vi "Main Display Console.vi"(8 "error in (no error)":errorcluster, 11 "Module_Refs":T2={"ModuleName"=enum."Controller", "Queue"=refnum, "user event"=refnum, "VI Refnum"=refnum, "ShowFP"=FALSE, "StatesTracking Enabled"=FALSE}) -> (0 "error out":errorcluster)   [LabVIEW 2019, in "DisplayConsole.lvlib"]
doc: "Main Module Template of the architecture. Use this as a template to integrate new independent processes into your application."
uses:
  DisplayConsole.lvlib
  Architecture/Typedefs/Enum_Module_Name.ctl
  Architecture/Architecture.lvlib
  Architecture/Typedefs/Message.ctl
  Architecture/Typedefs/Module References.ctl
  Typedefs/State Machine Data.ctl
  Architecture/Typedefs/Application Configuration.ctl
  Typedefs/Config.ctl
  Architecture/Modules/Module Template/SubVIs/Module Template Configuraton Extractor API.vi
  Architecture/Modules/Module Template/Typedefs/Config.ctl
  Architecture/Modules/Module Template/Module Template.lvlib
panel:
  in  "Display Console":T1
  in  "Stop App":bool
  out "Message":string
  in  "Stop Module":bool
  # "#Architecture\n\nPlace inside this box all visible data."
  # "DISPLAY CONSOLE"
  # "[Covers: SI1]"
  # "[Covers: UI3]"
  # "[Covers: UI1]"
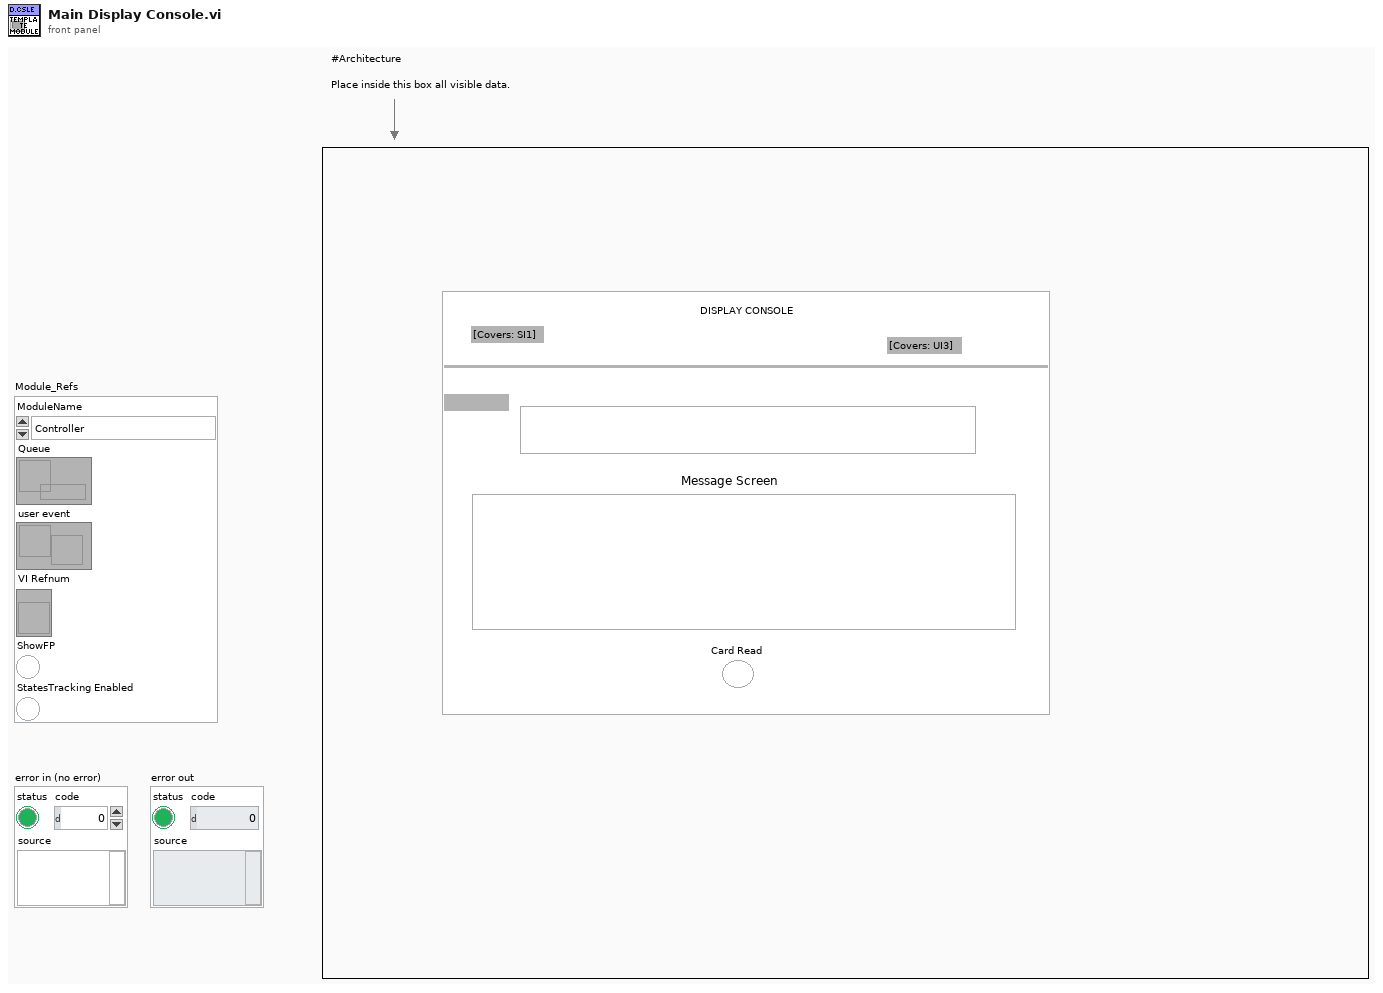
[diagram p1: front panel]
types:
  T1 = cluster{"Current Transaction":string, "Message Screen":string, "Card Read":bool}
  T2 = typedef "Architecture.lvlib/Module References.ctl" = cluster{"ModuleName":T3, "Queue":refnum<queue>, "user event":refnum<user-event>, "VI Refnum":refnum<vi>, "ShowFP":bool, "StatesTracking Enabled":bool}
  T3 = typedef "Architecture.lvlib/Enum_Module_Name.ctl" = enum16{"Configuration", "Error_Handler", "Log", "Database", "Controller", "User Console", "Display Console", "Sensor Interface"}
  T4 = typedef "DisplayConsole.lvlib/State Machine Data.ctl" = cluster{"Module_Refs":T2, "Response Data":variant, "Module Template Config":T5}
  T5 = typedef "DisplayConsole.lvlib/Config.ctl" = cluster{"Module Enabled":bool}
  T6 = enum32{"Invalid", "Standard", "Closed", "Hidden", "Minimized", "Maximized"}
  T7 = typedef "Architecture.lvlib/Module Template.lvlib/Config.ctl" = cluster{"Module Enabled":bool}
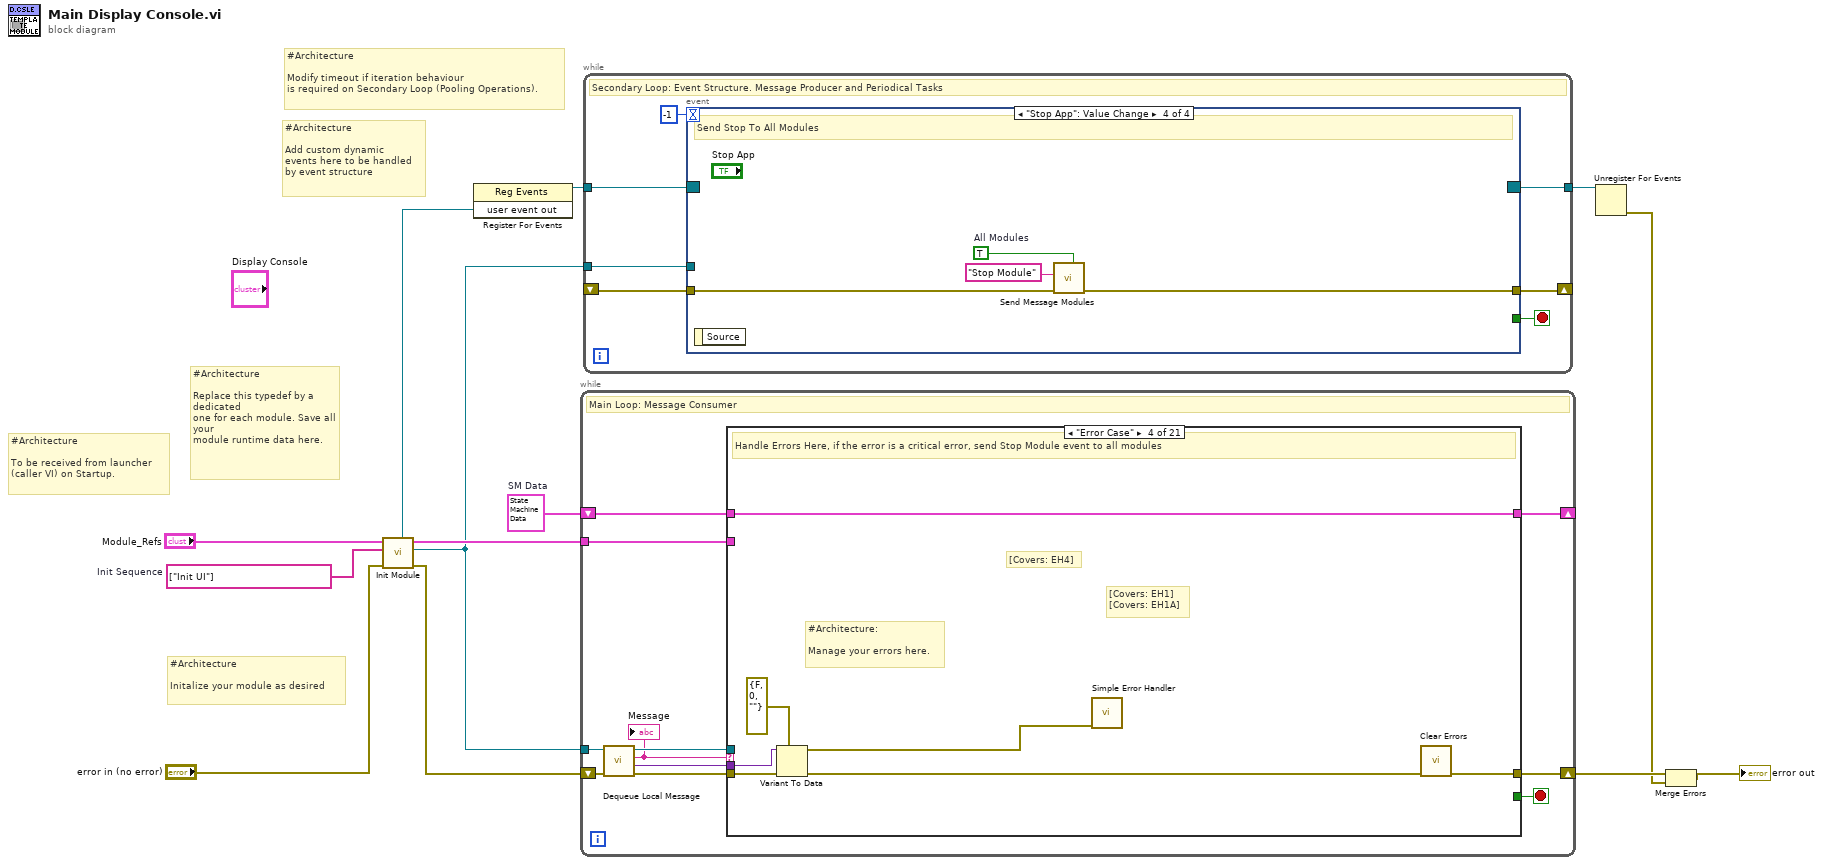
[diagram p0: block diagram]
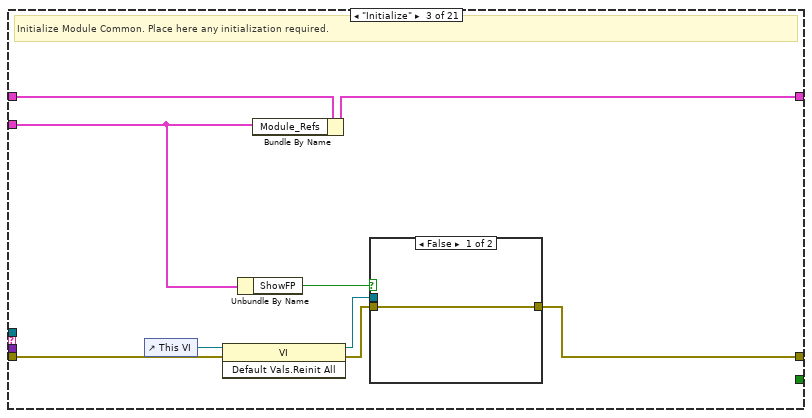
[diagram p4: hidden frame]
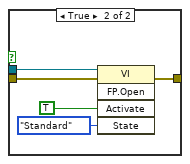
[diagram p5: hidden frame]
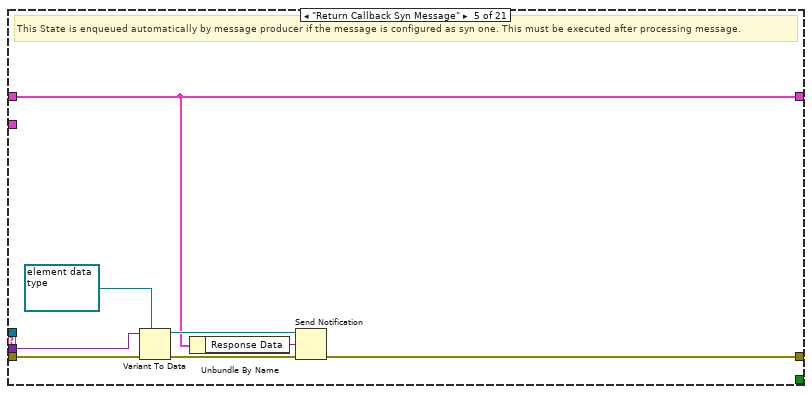
[diagram p6: hidden frame]
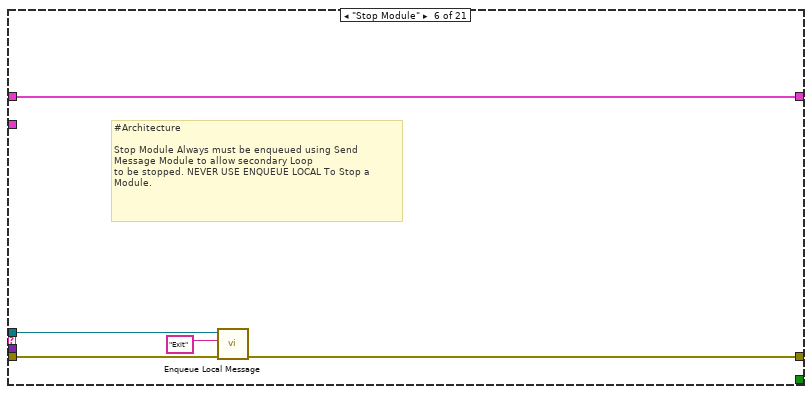
[diagram p7: hidden frame]
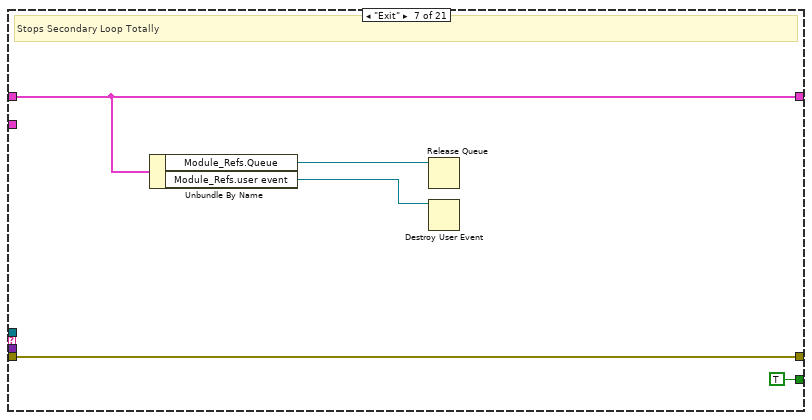
[diagram p8: hidden frame]
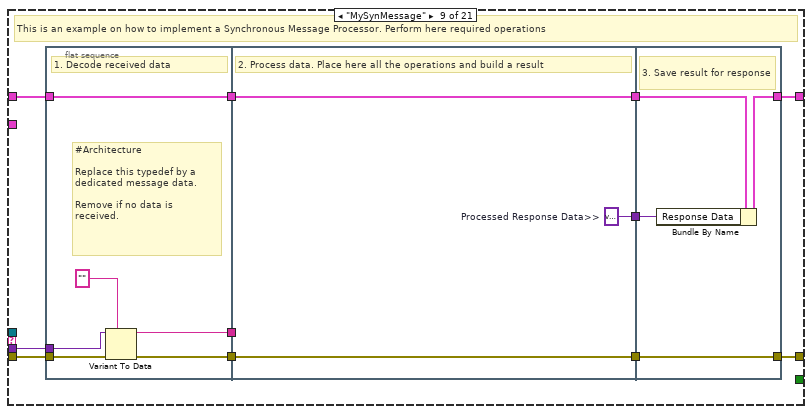
[diagram p10: hidden frame]
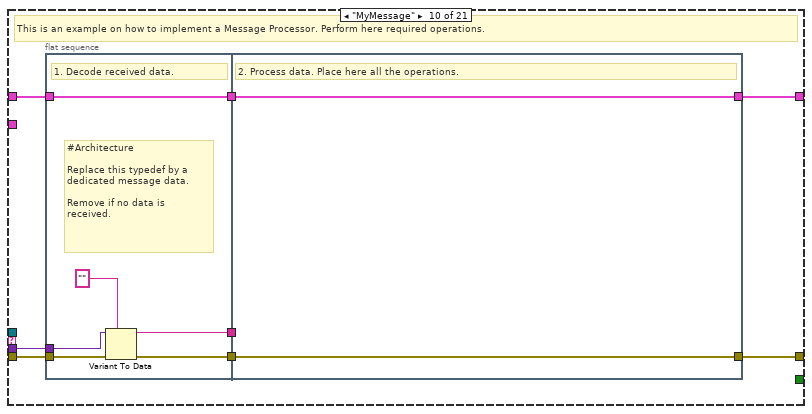
[diagram p11: hidden frame]
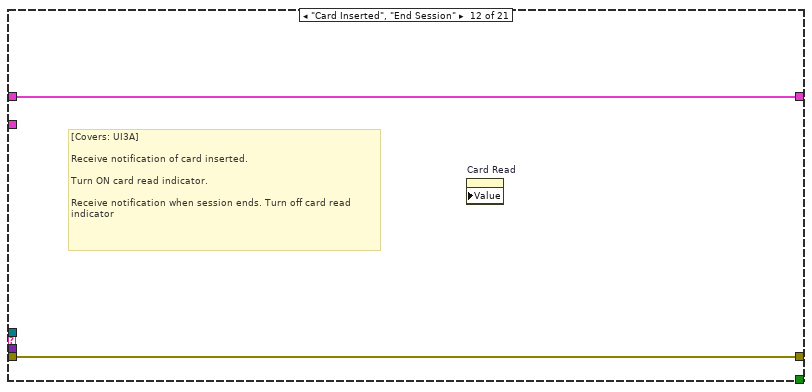
[diagram p13: hidden frame]
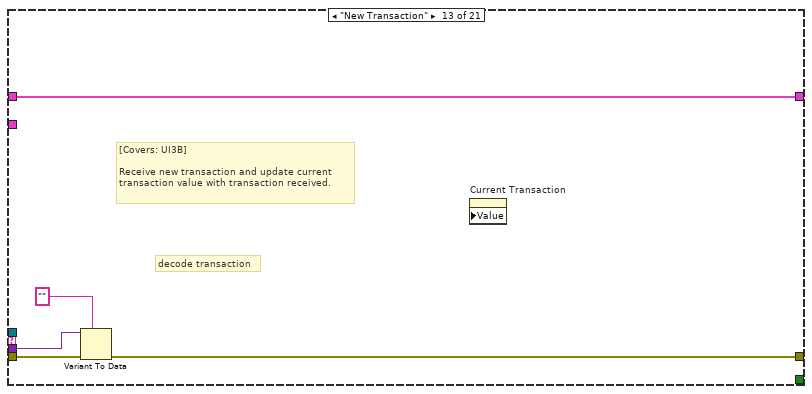
[diagram p14: hidden frame]
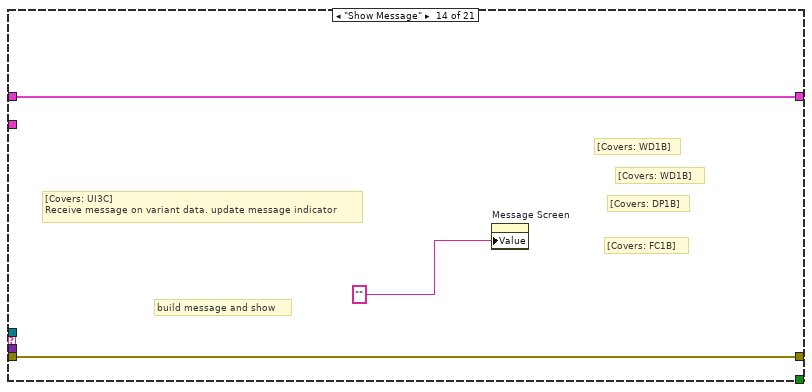
[diagram p15: hidden frame]
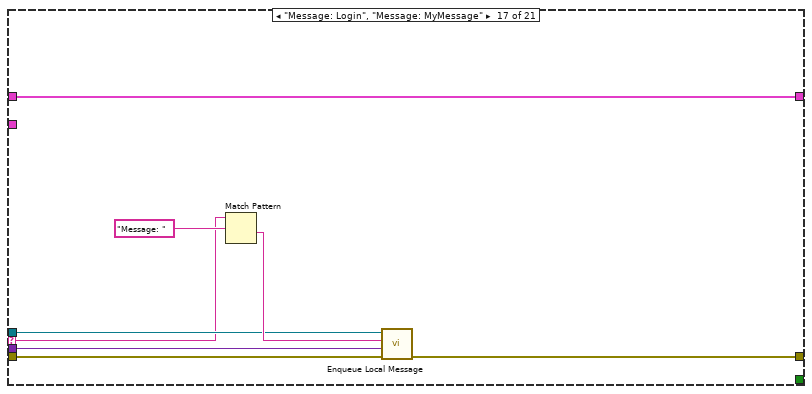
[diagram p18: hidden frame]
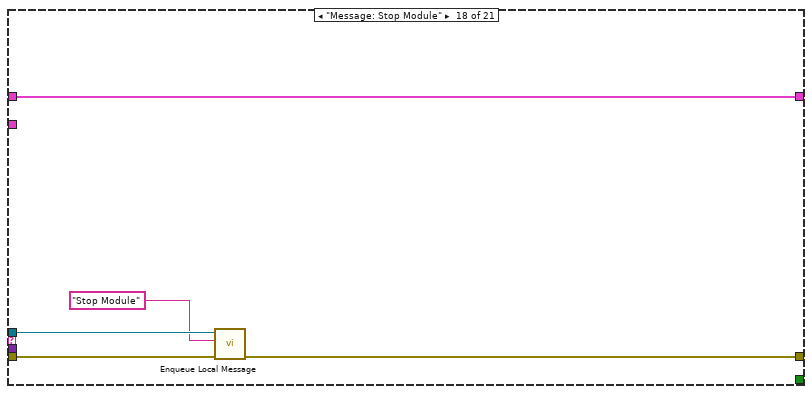
[diagram p19: hidden frame]
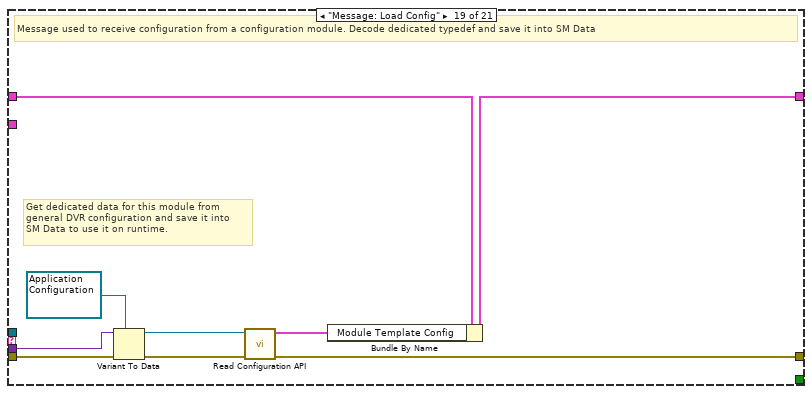
[diagram p20: hidden frame]
diagram:
  w10 = string[] ["Init UI"]  # Init Sequence
  w13 = T4 {"Module_Refs"={"ModuleName"=enum."Controller", "Queue"=refnum, "user event"=refnum, "VI Refnum"=refnum, "ShowFP"=FALSE, "StatesTracking Enabled"=FALSE}, "Response Data"=variant, "Module Template Config"={"Module Enabled"=FALSE}}  # SM Data
  # "#Architecture\n\nModify timeout if iteration behaviour \nis required on Secondary Loop (Pooling Operations)."
  # "#Architecture\n\nAdd custom dynamic \nevents here to be handled \nby event structure"
  # "#Architecture\n\nInitalize your module as desired"
  # "#Architecture\n\nTo be received from launcher \n(caller VI) on Startup."
  # "#Architecture\n\nReplace this typedef by a dedicated \none for each module. Save all your \nmodule runtime data here."
  n1 = call "Init Module.vi"("error in (no error)"="error in (no error)", "Init Sequence"=w10, "Module Refs"="Module_Refs") -> ("error out"=w12:errorcluster, "queue out"=w1:refnum<queue>, "Module Refs Out"=w3:T2, "user event out"=w2:refnum<user-event>)  [unwired: 5 in]
  n2 = register-events(w2) -> (reference out=w9:refnum<event-registration>)  [unwired: 2 in, 1 out]
  n3 = while {
    shift-right: [w23] -> _
    shift-left: w13 -> [w24]
    shift-right: [w22] -> w7
    shift-left: w12 -> [w20]
    tunnel: w1 -> [w21]
    tunnel: w3 -> [w14]
    stop <- w15 stop-if-true
    # "Main Loop: Message Consumer"
    n4 = call "Dequeue Local Message.vi"("error in"=w20, "Msg queue in"=w21) -> ("error out"=w19:errorcluster, "Data"=w16:variant, "Message"=w17:string, "queue out"=w18:refnum<queue>)  [unwired: 6 in]
    "Message" <- w17
    n5 = case shown="\"Error Case\"" w17 {
      selector: w17 -> [_ _ _ _ _ _ _ _ _ _ _ _ _ _ _ _ w127 _ _ _ w159]
      tunnel: w24 -> [w26 w28 w37 w50 w52 w63 w66 w70 w81 w102 w112 w114 w119 w122 w124 w126 w134 w139 w148 w150 w164]
      tunnel: [w26 w28 w35 w50 w52 w63 w66 w70 w80 w95 w112 w114 w119 w122 w124 w126 w134 w139 w141 w150 w164] -> w23
      tunnel: w19 -> [w25 w27 w36 w49 w58 w62 w68 w69 w74 w98 w111 w113 w118 w121 w123 w125 w131 w138 w147 w149 w163]
      tunnel: [w25 w27 w31 w45 w57 w61 w68 w69 w79 w101 w111 w113 w117 w121 w123 w125 w128 w137 w142 w149 w153] -> w22
      tunnel: w18 -> [_ _ _ _ _ w60 _ _ _ _ _ _ _ _ _ _ w129 w136 _ _ w160]
      tunnel: w16 -> [_ _ _ w47 w55 _ _ _ w73 w97 _ _ w115 _ _ _ w130 _ w146 _ w161]
      tunnel: [_ _ _ _ _ _ TRUE _ _ _ _ _ _ _ _ _ _ _ _ _ _] -> w15
      tunnel: w14 -> [_ _ w34 _ _ _ _ _ _ _ _ _ _ _ _ _ _ _ _ _ _]
      frame "--------State Machine Arquitechture Operations--------" {
      }
      frame "Idle", Default {
        # "Use this state to make iterations if required."
      }
      frame "Initialize" {
        # "Initialize Module Common. Place here any initialization required."
        n6 = control-ref of="This VI"() -> (w29:refnum<vi>)
        n7 = invoke class="VI" method="Default Vals.Reinit All"(reference=w29, error in=w36) -> (reference out=w32:refnum<vi>, error out=w33:errorcluster)  [unwired: 1 in, 1 out]
        n8 = Unbundle By Name(w34) -> ("ShowFP"=w30:bool)
        n9 = Bundle By Name(cluster=w37, "Module_Refs"=w34) -> (w35:T4)
        n10 = case shown="False" w30 {
          tunnel: w33 -> [w38 w43]
          tunnel: [w38 w42] -> w31
          tunnel: w32 -> [_ w41]
          frame False {
          }
          frame True {
            n11 = invoke class="VI" method="FP.Open"(reference=w41, error in=w43, "Activate"=TRUE ("Activate?"), "State"=T6."Standard") -> (error out=w42:errorcluster)  [unwired: 1 in, 4 out]
          }
        }
      }
      frame "Error Case" {
        # "[Covers: EH4]"
        # "[Covers: EH1] \n[Covers: EH1A]"
        # "#Architecture: \n\nManage your errors here."
        # "Handle Errors Here, if the error is a critical error, send Stop Module event to all modules"
        n12 = Variant To Data(error in=w49, type=errorcluster {"status"=FALSE, "code"=0, "source"=""} ("error constant"), Variant=w47) -> (data=w44:errorcluster, error out=w48:errorcluster)
        n13 = call <vilib>:"Simple Error Handler.vi"("error in (no error)"=w44) -> ()  [unwired: 4 in, 5 out]
        n14 = call <vilib>:"Clear Errors.vi"("error in (no error)"=w48) -> ("error out"=w45:errorcluster)  [unwired: 5 in, 1 out]
      }
      frame "Return Callback Syn Message" {
        # "This State is enqueued automatically by message producer if the message is configured as syn one. This must be executed after processing message."
        n15 = Variant To Data(error in=w58, type=refnum<notifier> refnum ("notifier out"), Variant=w55) -> (data=w53:refnum<notifier>, error out=w56:errorcluster)
        n16 = Unbundle By Name(w52) -> ("Response Data"=w51:variant)
        n17 = Send Notification(notification=w51, notifier=w53, error in (no error)=w56) -> (error out=w57:errorcluster)  [unwired: 1 out]
      }
      frame "Stop Module" {
        # "#Architecture\n\nStop Module Always must be enqueued using Send Message Module to allow secondary Loop\nto be stopped. NEVER USE ENQUEUE LOCAL To Stop a Module."
        n18 = call "Enqueue Local Message.vi"("error in"=w62, "Message"="Exit", "Msg queue in"=w60) -> ("error out"=w61:errorcluster)  [unwired: 7 in, 1 out]
      }
      frame "Exit" {
        # "Stops Secondary Loop Totally"
        n19 = Unbundle By Name(w66) -> ("Module_Refs.Queue"=w65:refnum<queue>, "Module_Refs.user event"=w64:refnum<user-event>)
        n20 = Release Queue(queue=w65) -> ()  [unwired: 2 in, 3 out]
        n21 = Destroy User Event(user event=w64) -> ()  [unwired: 1 in, 1 out]
      }
      frame "--------------State Machine Custom States-------------" {
      }
      frame "MySynMessage" {
        # "This is an example on how to implement a Synchronous Message Processor. Perform here required operations"
        n22 = flat-sequence {
          tunnel: w74 -> [w85]
          tunnel: w81 -> [w87]
          tunnel: [w87] -> w78
          tunnel: [w83] -> w77
          tunnel: w73 -> [w84]
          tunnel: [w82] -> w72
          tunnel: w78 -> [w90]
          tunnel: w77 -> [w89]
          tunnel: [w90] -> w76
          tunnel: [w89] -> w75
          tunnel: w72 -> [_]
          tunnel: [w88] -> w71
          tunnel: [w93] -> w79
          tunnel: [w92] -> w80
          tunnel: w76 -> [w94]
          tunnel: w75 -> [w93]
          tunnel: w71 -> [w91]
          frame #0 {
            # "#Architecture\n\nReplace this typedef by a dedicated message data.\n\nRemove if no data is received."
            # "1. Decode received data"
            n23 = Variant To Data(error in=w85, type="", Variant=w84) -> (data=w82:string, error out=w83:errorcluster)
          }
          frame #1 {
            w88 = variant  # Processed Response Data>>
            # "2. Process data. Place here all the operations and build a result"
          }
          frame #2 {
            # "3. Save result for response"
            n24 = Bundle By Name(cluster=w94, "Response Data"=w91) -> (w92:T4)
          }
        }
      }
      frame "MyMessage" {
        # "This is an example on how to implement a Message Processor. Perform here required operations."
        n25 = flat-sequence {
          tunnel: w98 -> [w106]
          tunnel: w102 -> [w108]
          tunnel: [w108] -> w100
          tunnel: [w104] -> w99
          tunnel: w97 -> [w105]
          tunnel: [w103] -> w96
          tunnel: w100 -> [w109]
          tunnel: w99 -> [w110]
          tunnel: w96 -> [_]
          tunnel: [w110] -> w101
          tunnel: [w109] -> w95
          frame #0 {
            # "#Architecture\n\nReplace this typedef by a dedicated message data.\n\nRemove if no data is received."
            # "1. Decode received data."
            n26 = Variant To Data(error in=w106, type="", Variant=w105) -> (data=w103:string, error out=w104:errorcluster)
          }
          frame #1 {
            # "2. Process data. Place here all the operations."
          }
        }
      }
      frame "Init UI" {
        # "[Covers: IS2]\n\nPlace here all calls to property nodes to \ninitialize UI controls and Indicators.\n\n• Card Read indicator is OFF.\n• Current Transaction indicator display is blank.\n• Message Screen indicator displays the Welcome Message, as specified in\nTable 1."
      }
      frame "Card Inserted", "End Session" {
        # "[Covers: UI3A] \n\nReceive notification of card inserted. \n\nTurn ON card read indicator.\n\nReceive notification when session ends. Turn off card read \nindicator"
        n27 = property on="Card Read" class="Bool (strict)" props=["Value"]() -> ()  [unwired: 3 in, 2 out]
      }
      frame "New Transaction" {
        # "decode transaction"
        # "[Covers: UI3B] \n\nReceive new transaction and update current \ntransaction value with transaction received."
        n28 = Variant To Data(error in=w118, type="", Variant=w115) -> (error out=w117:errorcluster)  [unwired: 1 out]
        n29 = property on="Current Transaction" class="Str" props=["Value"]() -> ()  [unwired: 3 in, 2 out]
      }
      frame "Show Message" {
        # "[Covers: FC1B]"
        # "[Covers: WD1B]"
        # "[Covers: WD1B]"
        # "[Covers: DP1B]"
        # "build message and show"
        # "[Covers: UI3C] \nReceive message on variant data. update message indicator"
        n30 = property on="Message Screen" class="Str"("Value"="") -> ()  [unwired: 2 in, 2 out]
      }
      frame "Login" {
        # "[Covers: LO1B]"
        # "[Covers: ID1A] \n\nInit controls on Login"
      }
      frame "--------------Dynamic Events Messages----------------" {
      }
      frame "Message: Login", "Message: MyMessage" {
        n31 = Match Pattern(string=w127, regular expression="Message: ") -> (after substring=w132:string)  [unwired: 1 in, 3 out]
        n32 = call "Enqueue Local Message.vi"("error in"=w131, "Data"=w130, "Message"=w132, "Msg queue in"=w129) -> ("error out"=w128:errorcluster)  [unwired: 6 in, 1 out]
      }
      frame "Message: Stop Module" {
        n33 = call "Enqueue Local Message.vi"("error in"=w138, "Message"="Stop Module", "Msg queue in"=w136) -> ("error out"=w137:errorcluster)  [unwired: 7 in, 1 out]
      }
      frame "Message: Load Config" {
        # "Get dedicated data for this module from \ngeneral DVR configuration and save it into \nSM Data to use it on runtime."
        # "Message used to receive configuration from a configuration module. Decode dedicated typedef and save it into SM Data"
        n34 = Variant To Data(error in=w147, type=refnum<data-value> refnum ("data value reference"), Variant=w146) -> (data=w144:refnum<data-value>, error out=w143:errorcluster)
        n35 = call-poly "Read Configuration API.vi"("error constant"=w143, "General Config DVR In"=w144) -> ("error out"=w142:errorcluster, "Module Template Config"=w140:T7)  [unwired: 8 in]
        n36 = Bundle By Name(cluster=w148, "Module Template Config"=w140) -> (w141:T4)
      }
      frame "------------Synchronous Event Messages--------------" {
      }
      frame "SynMessage: MySynMessage" {
        # "Use this case as a handler for Synchronous messages. This state queues a message for the desired"
        n37 = call "Extract Synchronous Data.vi"("error in 2"=w163, "Variant"=w161) -> ("error in"=w162:errorcluster, "Data Out"=w156:variant, "notifier out"=w151:refnum<notifier>)  [unwired: 7 in]
        n38 = Match Pattern(string=w159, regular expression="SynMessage: ") -> (after substring=w157:string)  [unwired: 1 in, 3 out]
        n39 = call "Enqueue Local Message.vi"("error in"=w162, "Data"=w156, "Message"=w157, "Msg queue in"=w160) -> ("error out"=w155:errorcluster, "queue out"=w154:refnum<queue>)  [unwired: 6 in]
        n40 = call "Enqueue Local Message.vi"("error in"=w155, "Data"=w151, "Message"="Return Callback Syn Message", "Msg queue in"=w154) -> ("error out"=w153:errorcluster)  [unwired: 6 in, 1 out]
      }
    }
  }
  n41 = while {
    tunnel: w9 -> [w171]
    tunnel: w1 -> [w168]
    tunnel: [w167] -> w8
    shift-right: [w165] -> _
    shift-left: _ -> [w166]
    stop <- w169 stop-if-true
    # "Secondary Loop: Event Structure. Message Producer and Periodical Tasks"
    n42 = event shown="[3] \"Stop App\": Value Change" {
      selector: w171 -> [_ _ _ _]
      dyn-events: [_ _ _ _] -> w167
      timeout: -1 -> [_ _ _ _]
      tunnel: [FALSE w180 TRUE _] -> w169
      tunnel: w168 -> [_ w185 w187 _]
      tunnel: w166 -> [w172 w184 w190 w192]
      tunnel: [w172 w183 w188 w191] -> w165
      event Timeout {
        n43 = event-data() -> ()  [unwired: 1 in, 1 out]
      }
      event User Event {
        # "Send message to local queue. \n(Message Consumer)"
        # "Processes an external event and enqueues a message to the local queue. It can be synchronous (with response) or NOT."
        n44 = event-data() -> ("syn"=w177:bool, "Message"=w179:string, "Data"=w182:variant)  [unwired: 1 in]
        n45 = Select(t="SynMessage: " ("string"), s=w177, f="Message: " ("string")) -> (s? t:f=w174:string)
        n46 = Concatenate Strings(w174, w179) -> (w181:string)
        n47 = call "Enqueue Local Message.vi"("error in"=w184, "Data"=w182, "Message"=w181, "Msg queue in"=w185) -> ("error out"=w183:errorcluster)  [unwired: 6 in, 1 out]
        n48 = Equal?(x=w179, y="Stop Module") -> (x = y?=w180:bool)
      }
      event "Stop Module": Value Change {
        n49 = event-data() -> ()  [unwired: 1 in, 1 out]
        n50 = call "Enqueue Local Message.vi"("error in"=w190, "Message"="Stop Module", "Msg queue in"=w187) -> ("error out"=w188:errorcluster)  [unwired: 7 in, 1 out]
      }
      event "Stop App": Value Change {
        w194 = TRUE  # All Modules
        # "Send Stop To All Modules"
        n51 = event-data() -> ()  [unwired: 1 in, 1 out]
        n52 = call "Send Message Modules.vi"("All Modules"=w194, "Error In"=w192, "Message"="Stop Module") -> ("error in (no error)"=w191:errorcluster)  [unwired: 8 in]
      }
    }
  }
  n53 = Unregister For Events(event registration refnum=w8) -> (error out=w6:errorcluster)  [unwired: 1 in]
  n54 = Merge Errors(w7, w6) -> (→"error out":errorcluster)
